vi "array -- first zero.vi"(11 "temperatures":dbl[](array[numeric])=[10.0, 20.0, 56.0, 92.0, 120.0, 183.0, 194.0, 310.0]) -> (2 "element index":i32, 3 "zero found":bool)   [LabVIEW 2010]
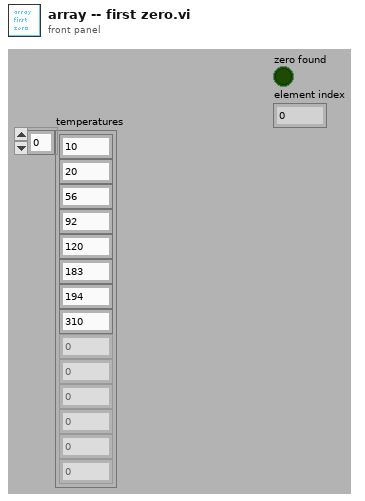
[diagram p1: front panel]
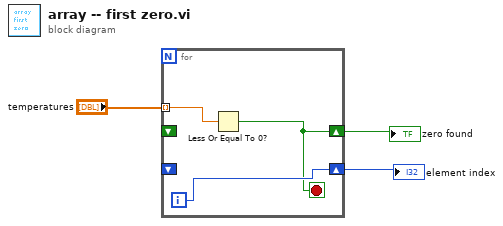
[diagram p0: block diagram]
diagram:
  n1 = for {
    tunnel: "temperatures" -> [w6] mode=indexing
    shift-right: [w5] -> w2
    shift-left: _ -> [_]
    shift-right: [w4] -> w1
    shift-left: _ -> [_]
    i -> [w5]
    stop <- w4 stop-if-true
    n2 = Less Or Equal To 0?(x=w6) -> (x <= 0?=w4:bool)
  }
  "zero found" <- w1
  "element index" <- w2
